vi "Write File to Server.vi"(8 "error in (no error)":errorcluster, 10 "Local FilePath":path, 11 "FTP in":refnum<class "FTP.lvclass">) -> (0 "error out":errorcluster, 3 "FTP out":refnum<class "FTP.lvclass">)   [LabVIEW 2017, in "FTP_UpgradeCSMF.lvlib" / "FTP.lvclass"]
uses:
  FTP.lvclass
  FTP.lvclass/FTP.ctl
  controls/File Transfer Status.ctl
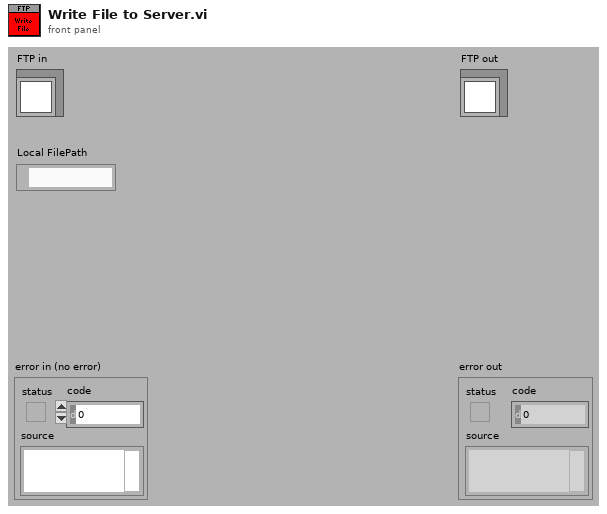
[diagram p1: front panel]
types:
  T1 = typedef "FTP_UpgradeCSMF.lvlib/FTP.lvclass/File Transfer Status.ctl" = cluster{"File Name":string, "Percent Complete":u8, "File Size (in bytes)":i64, "Bytes Sent or Rcvd":i64}
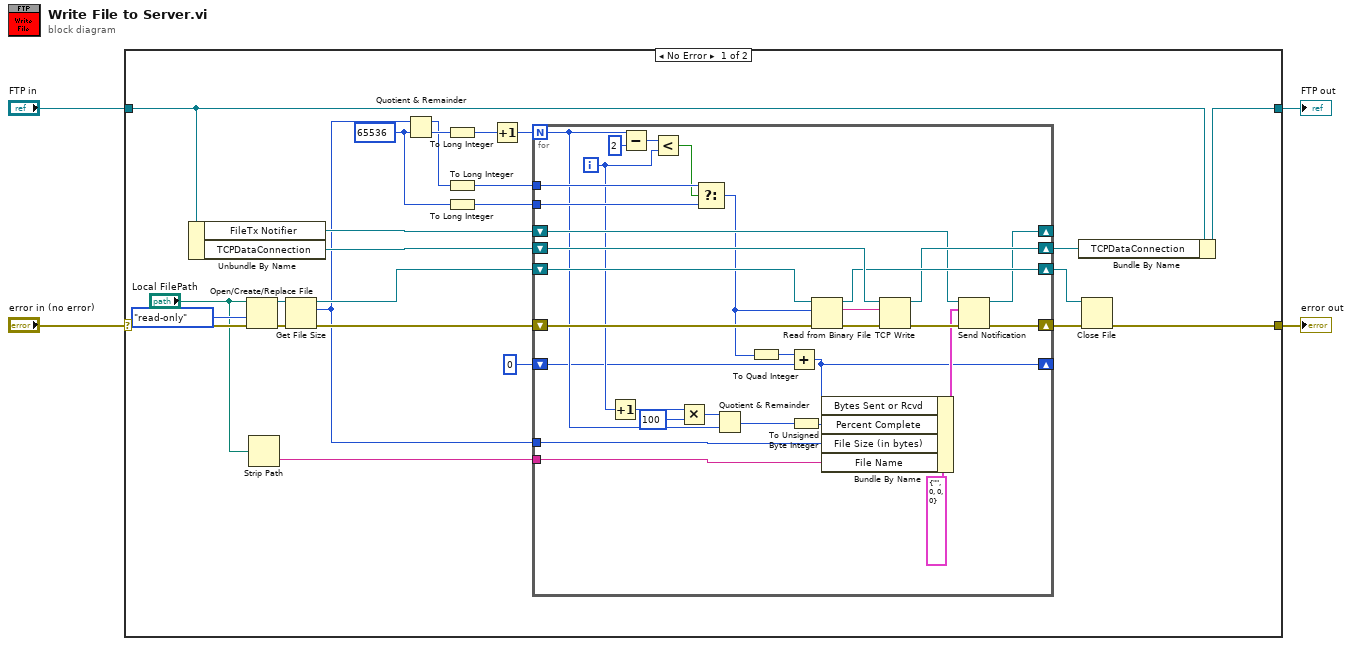
[diagram p0: block diagram]
diagram:
  n1 = case shown="No Error" "error in (no error)" {
    selector: "error in (no error)" -> [w24 w62]
    tunnel: [w17 w62] -> w3
    tunnel: [w12 w61] -> w1
    tunnel: "FTP in" -> [w23 w61]
    frame No Error {
      w19 = i64 65536 ("y")
      n2 = Unbundle By Name(w23) -> ("FileTx Notifier"=w9:refnum<notifier>, "TCPDataConnection"=w22:refnum<k5>)
      n3 = Open/Create/Replace File(file path (use dialog)="Local FilePath", error in=w24, access (0:read/write)=enum16{"read/write", "read-only", "write-only"}."read-only") -> (refnum out=w28:refnum<file>, error out=w29:errorcluster)  [unwired: 3 in, 1 out]
      n4 = Strip Path(path="Local FilePath") -> (name=w7:string)  [unwired: 1 out]
      n5 = Get File Size(file=w28, error in=w29) -> (refnum out=w25:refnum<file>, size (in bytes)=w6:i64, 0:w26:errorcluster)
      n6 = Quotient & Remainder(x=w6, y=w19) -> (x-y*floor(x/y)=w14:i64, floor(x/y)=w27:i64)
      n7 = To Long Integer(number=w27) -> (32bit integer=w16:i32)
      n8 = To Long Integer(number=w14) -> (32bit integer=w13:i32)
      n9 = To Long Integer(number=w19) -> (32bit integer=w18:i32)
      n10 = Increment(x=w16) -> (x+1=w15:i32)
      n11 = for {
        N: w15 -> [w37]
        shift-right: [w47] -> w21
        shift-left: w26 -> [w60]
        shift-right: [w56] -> w20
        shift-left: w25 -> [w59]
        shift-right: [w55] -> w11
        shift-left: w22 -> [w57]
        tunnel: w18 -> [w50]
        tunnel: w13 -> [w51]
        shift-right: [w46] -> _
        shift-left: w9 -> [w45]
        tunnel: w7 -> [w43]
        tunnel: w6 -> [w34]
        shift-right: [w32] -> _
        shift-left: i64 0 -> [w33]
        i -> [w41]
        n12 = Increment(x=w41) -> (x+1=w39:i32)
        n13 = Subtract(x=w37, y=2) -> (x-y=w52:i32)
        n14 = Less?(x=w52, y=w41) -> (x < y?=w49:bool)
        n15 = Multiply(x=w39, y=100) -> (x*y=w38:i32)
        n16 = Select(t=w51, s=w49, f=w50) -> (s? t:f=w31:i32)
        n17 = Quotient & Remainder(x=w38, y=w37) -> (floor(x/y)=w36:i32)  [unwired: 1 out]
        n18 = To Quad Integer(1:w31) -> (0:w30:i64)
        n19 = Add(x=w30, y=w33) -> (x+y=w32:i64)
        n20 = To Unsigned Byte Integer(number=w36) -> (unsigned 8bit integer=w35:u8)
        n21 = Read from Binary File(8:w60, 10:w31, 11:w59) -> (0:w58:errorcluster, 2:w54:string, 3:w56:refnum<file>)  [unwired: 3 in, 1 out]
        n22 = Bundle By Name(cluster=T1 {"File Name"="", "Percent Complete"=0, "File Size (in bytes)"=0, "Bytes Sent or Rcvd"=0} ("notification"), "Bytes Sent or Rcvd"=w32, "Percent Complete"=w35, "File Size (in bytes)"=w34, "File Name"=w43) -> (w42:T1)
        n23 = TCP Write(connection ID=w57, data in=w54, error in (no error)=w58) -> (connection ID out=w55:refnum<k5>, error out=w48:errorcluster)  [unwired: 1 in, 1 out]
        n24 = Send Notification(notification=w42, notifier=w45, error in (no error)=w48) -> (notifier out=w46:refnum<notifier>, error out=w47:errorcluster)
      }
      n25 = Bundle By Name(cluster=w23, "TCPDataConnection"=w11) -> (w12:refnum<class "FTP.lvclass">)
      n26 = Close File(refnum=w20, error in=w21) -> (error out=w17:errorcluster)  [unwired: 1 out]
    }
    frame Error {
    }
  }
  "error out" <- w3
  "FTP out" <- w1
